vi "Get Actor Identifier from Actor.vi"(11 "Actor in":refnum<class "Actor.lvclass">) -> (2 "Valid Enqueuer?":bool, 3 "Actor ID string out":string)   [LabVIEW 2020, in "Utility.lvlib"]
doc: "Get the unique ID from 'Message Enqueuer'."
uses:
  Utility.lvlib
  PPL/HDH.Actor Framework.Core.Actor.lvlibp/1abvi3w/vi.lib/ActorFramework/Actor/Actor.lvclass
  PPL/HDH.Actor Framework.Core.Actor.lvlibp/1abvi3w/vi.lib/ActorFramework/Actor/Read Self Enqueuer.vi
  Private/Private Actor/Private Actor.lvclass
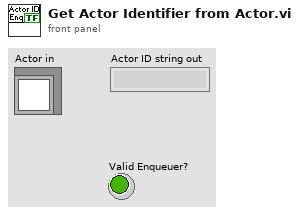
[diagram p1: front panel]
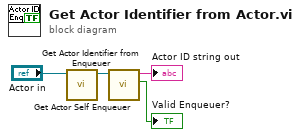
[diagram p0: block diagram]
diagram:
  n1 = call "Get Actor Self Enqueuer.vi"("Actor in"="Actor in") -> ("Self Enqueuer"=w3:refnum<class "Message Enqueuer.lvclass">)  [unwired: 10 in]
  n2 = call "Get Actor Identifier from Enqueuer.vi"("Message Enqueuer in"=w3) -> ("Valid Enqueuer?"=→"Valid Enqueuer?":bool, "Actor ID string out"=→"Actor ID string out":string)  [unwired: 9 in]
